vi "DrivePath-C.vi"(11 "Params":string[][](array[string])) -> ()   [LabVIEW 2020]
uses:
  Dawgma Programming Library/Controls/PurePursuit/PathFileData.ctl
  Dawgma Programming Library/Controls/PurePursuit/RobotNeededPathData.ctl
  Framework/Robot Global Data.vi
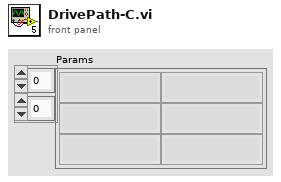
[diagram p1: front panel]
types:
  T1 = typedef "PathFileData.ctl" = cluster{"RobotNeeded":T2, "Meta":cluster{"Path (px)":cluster{i32, i32}[], "RobotWidth":dbl, "RobotLength":dbl, "CenterOfRotYOffset":dbl, "Roundedness":dbl, "StartingPositionPreset":u32, "PathName":string}}
  T2 = typedef "RobotNeededPathData.ctl" = cluster{"Path":cluster{dbl, dbl}[], "MaxVel":dbl, "MaxAccel":dbl, "Backwards?":bool, "PointSpacing":dbl, "LookaheadDist":dbl, "Speed/Curve":dbl, "SlowDistanceAtEnd":dbl, "SlowSpeed":dbl, "MaxDeAccel":dbl}
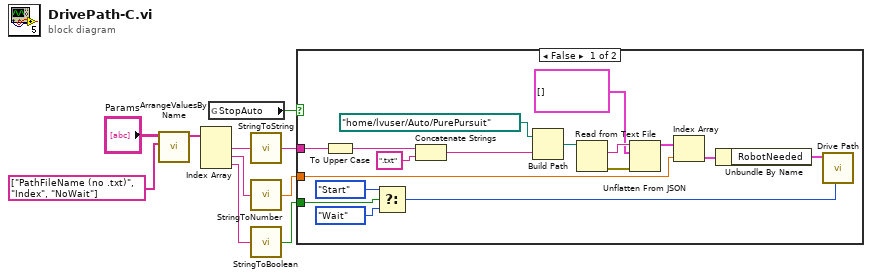
[diagram p0: block diagram]
diagram:
  n1 = call "ArrangeValuesByName.vi"("Names"=string[] ["PathFileName (no .txt)", "Index", "NoWait"], "Names/Values in"="Params") -> ("Values Out"=w4:string[])  [unwired: 9 in]
  n2 = Index Array(array=w4) -> (element #1=w3:string, element #2=w2:string, element #3=w1:string)  [unwired: 3 in]
  n3 = global read "Robot Global Data.vi" "StopAuto"() -> (w10:bool)
  n4 = call "StringToString.vi"("String"=w3) -> ("Output"=w7:string)
  n5 = call "StringToNumber.vi"("String"=w2) -> ("Output"=w8:dbl)
  n6 = call "StringToBoolean.vi"("String"=w1) -> ("Output"=w9:bool)
  n7 = case shown="False" w10 {
    tunnel: w9 -> [w15 _]
    tunnel: w8 -> [w13 _]
    tunnel: w7 -> [w12 _]
    frame False {
      n8 = To Upper Case(1:w12) -> (0:w11:string)
      n9 = Select(t=enum16{"Start", "Wait"}."Start" ("Synchronication"), s=w15, f=enum16{"Start", "Wait"}."Wait" ("Synchronication")) -> (s? t:f=w14:enum16{"Start", "Wait"})
      n10 = Concatenate Strings(w11, ".txt" ("string")) -> (w26:string)
      n11 = Build Path(base path=path "/home/lvuser/Auto/PurePursuit", name or relative path=w26) -> (appended path=w24:path)
      n12 = Read from Text File(file (use dialog)=w24) -> (text=w22:string, error out=w23:errorcluster)  [unwired: 3 in, 2 out]
      n13 = Unflatten From JSON(JSON string=w22, type and defaults=T1[] [], error in (no error)=w23) -> (value=w20:T1[])  [unwired: 4 in, 1 out]
      n14 = Index Array(array=w20, index=w13) -> (element=w19:T1)
      n15 = Unbundle By Name(w19) -> ("RobotNeeded"=w18:T2)
      n16 = call "Drive Path.vi"("Synchronication"=w14, "RobotNeededPathData"=w18) -> ()  [unwired: 9 in, 1 out]
    }
    frame True {
    }
  }
